vi "test_Open UDP connection using Clear Error node.vi"(8 "error in (no error)":errorcluster, 11 "TestCase in":refnum<class "Ethernet Protocol Tests.lvclass">) -> (0 "error out":errorcluster, 3 "TestCase out":refnum<class "Ethernet Protocol Tests.lvclass">)   [LabVIEW 2019, in "Ethernet Protocol Tests.lvclass"]
uses:
  Ethernet Protocol Tests.lvclass
  UDP/UDP.lvclass
  UDP/UDP.lvclass/UDP.ctl
  UDP/Data Access/Write Local IP Address.vi
  UDP/Data Access/Write Target IP Address.vi
  UDP/Data Access/Write Local Port.vi
  UDP/Data Access/Write Target Port.vi
  <vilib>/Utility/error.llb/Error Cluster From Error Code.vi
  Constants.vi
  <vilib>/ErrorRing/Error Ring.xnode
  <vilib>/addons/_JKI Toolkits/VI Tester/TestCase.llb/TestCase.lvclass
  C:/Program Files (x86)/National Instruments/LabVIEW 2019/vi.lib/addons/_JKI Toolkits/VI Tester/TestCase.llb/TestCase.lvclass
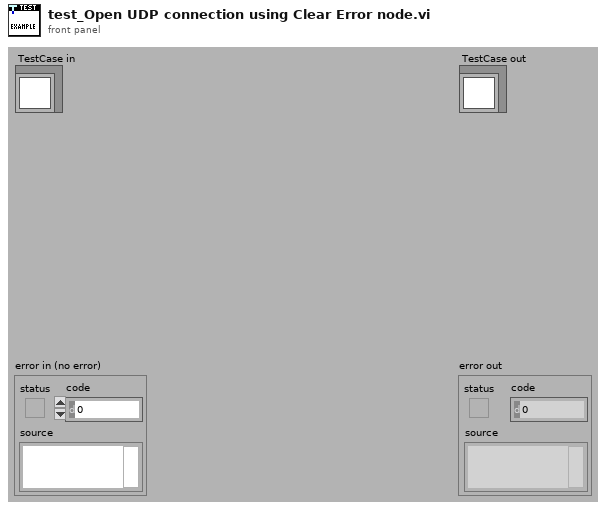
[diagram p1: front panel]
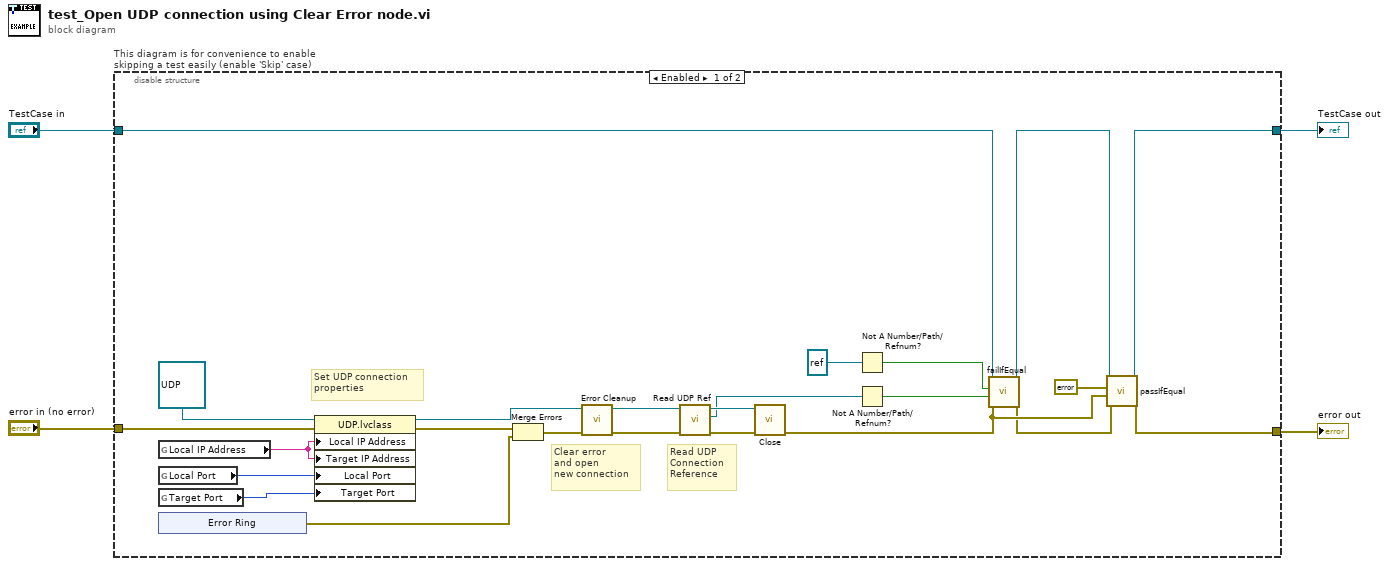
[diagram p0: block diagram]
diagram:
  n1 = disable-structure "This diagram is for convenience to enable skipping a test easily (enable 'Skip' case)" shown="Enabled" {
    disable-tunnel: "TestCase in" -> [w28 w37]
    disable-tunnel: [w7 w35] -> w1
    disable-tunnel: [w5 w36] -> w3
    disable-tunnel: "error in (no error)" -> [w26 w34]
    frame Enabled {
      # "Read UDP\nConnection \nReference"
      # "Clear error \nand open \nnew connection"
      # "Set UDP connection \nproperties"
      n2 = global read "Constants.vi" "Local IP Address"() -> (w13:string)
      n3 = global read "Constants.vi" "Local Port"() -> (w12:u16)
      n4 = global read "Constants.vi" "Target Port"() -> (w11:u16)
      n5 = xnode "Error Ring"() -> ("error out"=w23:errorcluster)
      n6 = property class="UDP.lvclass"(reference=refnum<class "UDP.lvclass"> refnum ("Protocols.lvlib:UDP.lvclass"), error in=w26, "Local IP Address"=w13, "Target IP Address"=w13, "Local Port"=w12, "Target Port"=w11) -> (reference out=w22:refnum<class "UDP.lvclass">, error out=w25:errorcluster)
      n7 = Merge Errors(w25, w23) -> (w24:errorcluster)
      n8 = call-dynamic "Error Cleanup.vi"("error in (no error)"=w24, "UDP in"=w22) -> ("error out"=w21:errorcluster, "UDP out"=w20:refnum<class "UDP.lvclass">)  [unwired: 8 in]
      n9 = call "Read UDP Ref.vi"("error in (no error)"=w21, "UDP in"=w20) -> ("error out"=w19:errorcluster, "UDP Ref"=w17:refnum<k16>, "UDP out"=w18:refnum<class "UDP.lvclass">)  [unwired: 7 in]
      n10 = call-dynamic "Close.vi"("error in (no error)"=w19, "UDP in"=w18) -> ("error out"=w10:errorcluster)  [unwired: 8 in, 1 out]
      n11 = Not A Number/Path/Refnum?(number/path/refnum=refnum<k16> refnum ("UDP Ref")) -> (NaN/Path/Refnum?=w14:bool)
      n12 = Not A Number/Path/Refnum?(number/path/refnum=w17) -> (NaN/Path/Refnum?=w16:bool)
      n13 = call-dynamic "failIfEqual.vi"("error in (no error)"=w10, "y"=w16, "x"=w14, "TestCase in"=w28) -> ("error out"=w9:errorcluster, "TestCase out"=w8:refnum<class "Ethernet Protocol Tests.lvclass">)  [unwired: 6 in]
      n14 = call-dynamic "passIfEqual.vi"("error in (no error)"=w9, "y"=w10, "x"=errorcluster {"status"=FALSE, "code"=0, "source"=""} ("error constant"), "TestCase in"=w8) -> ("error out"=w5:errorcluster, "TestCase out"=w7:refnum<class "Ethernet Protocol Tests.lvclass">)  [unwired: 6 in]
    }
    frame Disabled {
      # "skip test result while test is under development"
      n15 = call <vilib>:"skip.vi"("error in (no error)"=w34, "TestCase in"=w37) -> ("error out"=w36:errorcluster, "TestCase out"=w35:refnum<class "Ethernet Protocol Tests.lvclass">)  [unwired: 8 in]
    }
  }
  "error out" <- w3
  "TestCase out" <- w1
